vi "set up parameters Real.vi"(0 "i initial":dbl, 1 "i final":dbl=10.0, 2 "X-point":cdb=0.6+6.0i, 3 "theta":ext=1.47, 4 "Mag":dbl=1.0, 5 "Initial":dbl[](array[numeric])=[-0.05, 0.05, 0.3] format="%_3g") -> (8 "Skeleton":cluster{"B+i Vsg":cdb[]}[](array[cluster])=[{"B+i Vsg"=[-0.05+0.0i, 0.575+5.5i, 0.625+6.5i, 1.0863636363636364+10.0i]}, {"B+i Vsg"=[0.05+0.0i, 0.575+5.5i, 0.625+6.5i, 1.0045454545454544+10.0i]}, {"B+i Vsg"=[0.3+0.0i, 0.575+5.5i, 0.625+6.5i, 0.7999999999999999+10.0i]}] {"B+i Vsg" format="%_3g"}, 10 "XY Graph":cluster{dbl[], dbl[]}[](graph)=[{[0.0, 5.5, 6.5, 10.0], [-0.05, 0.575, 0.625, 1.0863636363636364]}, {[0.0, 5.5, 6.5, 10.0], [0.05, 0.575, 0.625, 1.0045454545454544]}, {[0.0, 5.5, 6.5, 10.0], [0.3, 0.575, 0.625, 0.7999999999999999]}])   [LabVIEW 2016]
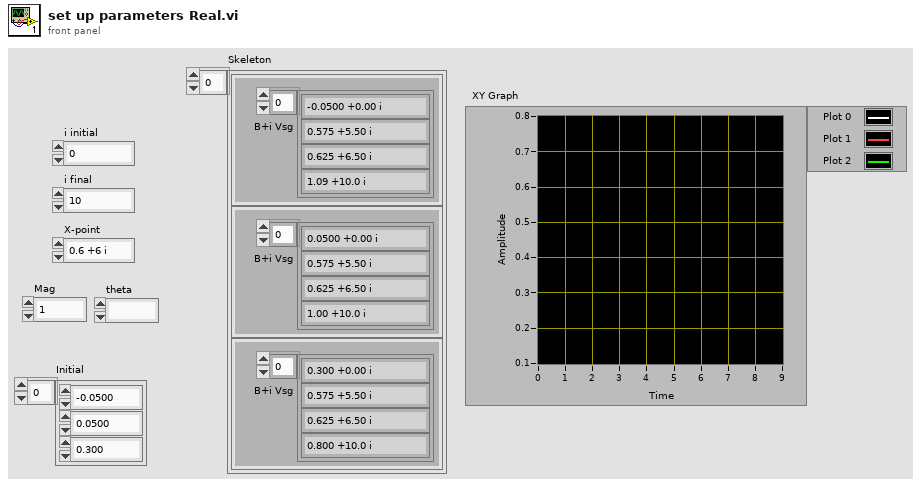
[diagram p1: front panel]
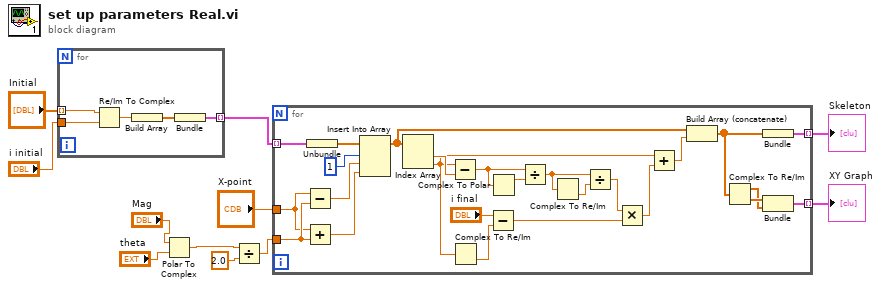
[diagram p0: block diagram]
diagram:
  n1 = for {
    tunnel: "Initial" -> [w15] mode=indexing
    tunnel: "i initial" -> [w16]
    tunnel: [w12] -> w6 mode=indexing
    n2 = Re/Im To Complex(1:w16, 2:w15) -> (0:w14:cdb)
    n3 = Build Array(w14) -> (w13:cdb[])
    n4 = Bundle(w13) -> (w12:cluster{cdb[]})  [unwired: 1 in]
  }
  n5 = Polar To Complex(1:"theta", 2:"Mag") -> (0:w1:cxt)
  n6 = Divide(x=w1, y=2.0) -> (x/y=w4:cxt)
  n7 = for {
    tunnel: "X-point" -> [w19]
    tunnel: w6 -> [w40] mode=indexing
    tunnel: [w38] -> w10 mode=indexing
    tunnel: [w23] -> w9 mode=indexing
    tunnel: w4 -> [w20]
    n8 = Subtract(x=w19, y=w20) -> (x-y=w18:cxt)
    n9 = Add(x=w19, y=w20) -> (x+y=w17:cxt)
    n10 = Unbundle(w40) -> (w39:cdb[])
    n11 = Insert Into Array(array=w39, index=1, new element #1=w18, new element #2=w17) -> (w26:cdb[])
    n12 = Index Array(array=w26) -> (element #1=w37:cdb, element #2=w28:cdb)  [unwired: 2 in]
    n13 = Subtract(x=w28, y=w37) -> (x-y=w35:cdb)
    n14 = Complex To Re/Im(x + iy=w28) -> (y=w33:dbl)  [unwired: 1 out]
    n15 = Subtract(x="i final", y=w33) -> (x-y=w30:dbl)
    n16 = Complex To Polar(r * e^(i*theta)=w35) -> (r=w36:dbl)  [unwired: 1 out]
    n17 = Divide(x=w35, y=w36) -> (x/y=w34:cdb)
    n18 = Complex To Re/Im(x + iy=w34) -> (y=w25:dbl)  [unwired: 1 out]
    n19 = Divide(x=w34, y=w25) -> (x/y=w31:cdb)
    n20 = Multiply(x=w31, y=w30) -> (x*y=w29:cdb)
    n21 = Add(x=w28, y=w29) -> (x+y=w27:cdb)
    n22 = Build Array (concatenate)(w26, w27) -> (w24:cdb[])
    n23 = Complex To Re/Im(x + iy=w24) -> (x=w21:dbl[], y=w22:dbl[])
    n24 = Bundle(w24) -> (w38:cluster{cdb[]})  [unwired: 1 in]
    n25 = Bundle(w22, w21) -> (w23:cluster{dbl[], dbl[]})  [unwired: 1 in]
  }
  "Skeleton" <- w10
  "XY Graph" <- w9
